vi "Set Key Focus.vi"(8 "error in (no error)":errorcluster, 10 "Key Focus":bool, 11 "Abstract Key Focus Msg in":refnum<class "Abstract Key Focus Msg.lvclass">) -> (0 "error out":errorcluster, 3 "Abstract Key Focus Msg out":refnum<class "Abstract Key Focus Msg.lvclass">)   [LabVIEW 2013, in "Create Project Model.lvlib" / "Abstract Key Focus Msg.lvclass"]
uses:
  Abstract Key Focus Msg.lvclass
  Abstract Key Focus Msg.lvclass/Abstract Key Focus Msg.ctl
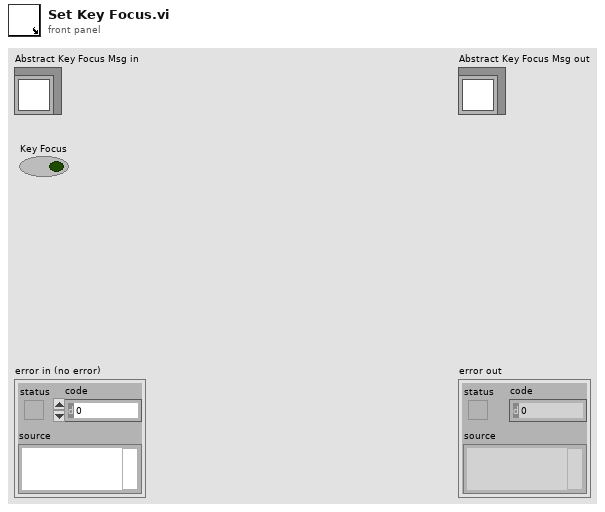
[diagram p1: front panel]
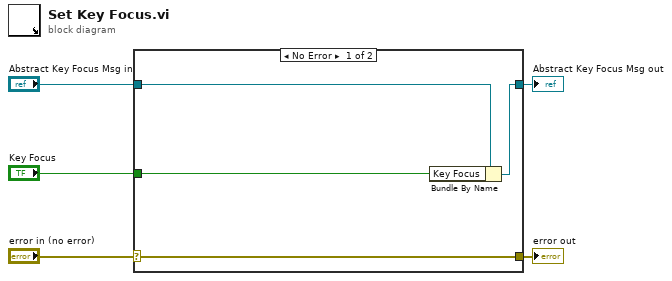
[diagram p0: block diagram]
diagram:
  n1 = case shown="No Error" "error in (no error)" {
    selector: "error in (no error)" -> [w9 w10]
    tunnel: [w9 w10] -> w4
    tunnel: [w7 w11] -> w2
    tunnel: "Abstract Key Focus Msg in" -> [w8 w11]
    tunnel: "Key Focus" -> [w6 _]
    frame No Error {
      n2 = Bundle By Name(cluster=w8, "Key Focus"=w6) -> (w7:refnum<class "Abstract Key Focus Msg.lvclass">)
    }
    frame Error {
    }
  }
  "error out" <- w4
  "Abstract Key Focus Msg out" <- w2
